vi "Connection.vi"(9 "전송":bool, 10 "데이터":string) -> ()   [LabVIEW 2020]
uses:
  <vilib>/Platform/TimedLoop/XDataNode/timing_clust.ctl
  <vilib>/Platform/TimedLoop/XDataNode/nitl_modes.ctl
  <vilib>/Platform/TimedLoop/XDataNode/wakeup.ctl
  WebSockets/WebSocket/WebSocket.lvclass/WebSocket.ctl
  WebSockets/WebSocket Server/WebSocket Server.lvclass/WebSocket Server.ctl
  WebSockets/WebSocket/Read Return Headers.vi
  WebSockets/WebSocket Server/Read Request URI.vi
  WebSockets/WebSocket Server/WebSocket Server.lvclass
  var.vi
  <vilib>/Platform/TimedLoop/XDataNode/XDataNode.xnode
  Sockets/VISA TCP Listener/VISA TCP Listener.lvclass
  <vilib>/Platform/TimedLoop/XDataNode/XDNodeRunTimeDep.lvlib
panel:
  out "데이터_자동":string
  in  "Stop":bool
  out "수신된 데이터":string
  out "HTTP Headers":variant
  out "Request URI":string
  # "소켓통신을 전담하는 subVI"
  # "2017243031 최주홍"
  # "수동으로 전송하는 용도"
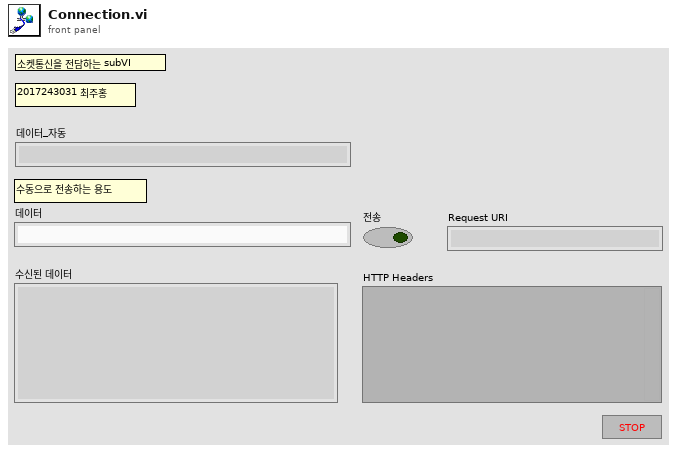
[diagram p1: front panel]
types:
  T1 = typedef "XDNodeRunTimeDep.lvlib/timing_clust.ctl" = cluster{"Expected End [f-1]":u64, "Actual End [f-1]":u64, "Finished Late? [f-1]":bool, "Expected End [i-1]":u64, "Actual End [i-1]":u64, "Finished Late? [i-1]":bool, "Expected Start [i]":u64, "Actual Start [i]":u64, "Expected Start [f]":u64, "Actual Start [f]":u64, "Source Name":string, "Structure Name":string, "Period":i64, "Deadline":i64, "Offset":i64, "Start":i64, "Priority":i32, "Timeout":i32, "Mode":T2, "Wakeup Reason":T3, "Error":errorcluster, "Source Type":string, "Secondary Source Type":string, "Global End Time":u64, "Global Start Time":u64, "Frame Duration":u64, "Iteration Duration":u64, "Assigned CPU":i32, "I/O Scan Engine Mode":u32}
  T2 = typedef "XDNodeRunTimeDep.lvlib/nitl_modes.ctl" = enum32{"No Change", "Process missed periods, maintain original phase", "Discard missed periods, maintain original phase", "Process missed periods, ignore original phase", "Discard missed periods, ignore original phase"}
  T3 = typedef "XDNodeRunTimeDep.lvlib/wakeup.ctl" = enum32{"Normal", "Aborted", "Asynchronous wakeup", "Timing source error", "Timed loop error", "Timeout"}
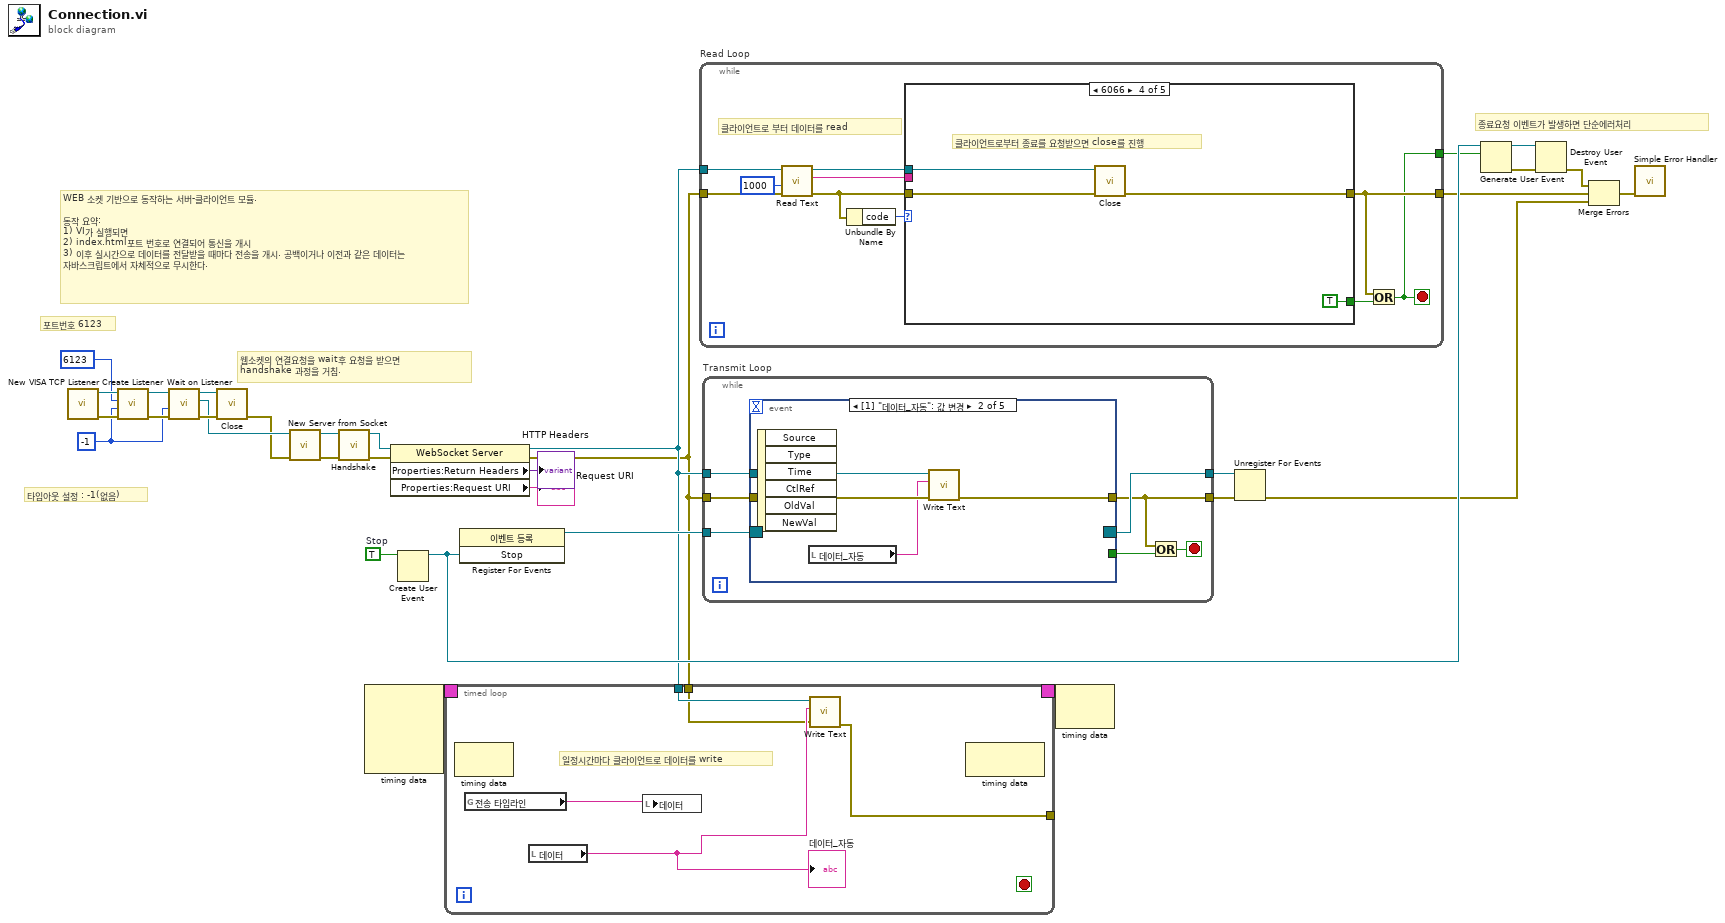
[diagram p0: block diagram]
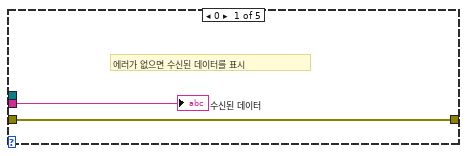
[diagram p2: hidden frame]
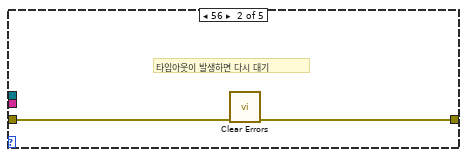
[diagram p3: hidden frame]
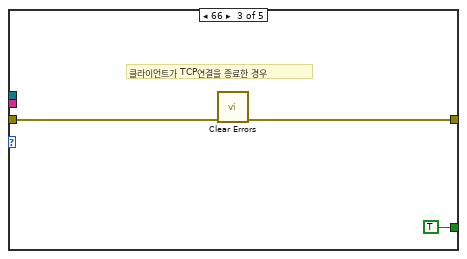
[diagram p4: hidden frame]
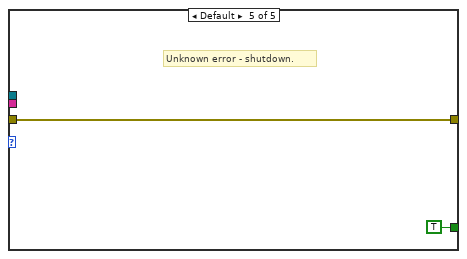
[diagram p5: hidden frame]
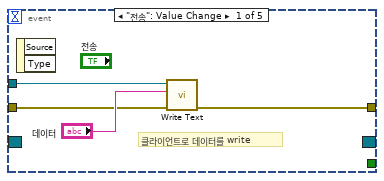
[diagram p6: hidden frame]
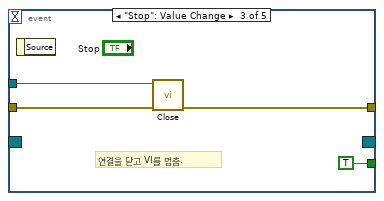
[diagram p7: hidden frame]
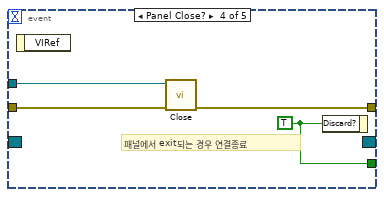
[diagram p8: hidden frame]
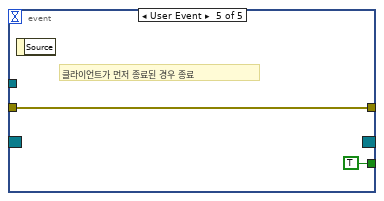
[diagram p9: hidden frame]
diagram:
  w31 = TRUE  # Stop
  w7 = -1 ("timeout ms (25000)")
  # "타임아웃 설정 : -1(없음)"
  # "종료요청 이벤트가 발생하면 단순에러처리"
  # "WEB 소켓 기반으로 동작하는 서버-클라이언트 모듈.\n\n동작 요약:\n1) VI가 실행되면\n2) index.html포트 번호로 연결되어 통신을 개시\n3) 이후 실시간으로 데이터를 전달받을 때마다 전송을 개시. 공백이거나 이전과 같은 데이터는 자바스크립트에서 자체적으로 무시한다."
  # "웹소켓의 연결요청을 wait후 요청을 받으면\nhandshake 과정을 거침."
  # "포트번호 6123"
  n1 = call "New VISA TCP Listener.vi"() -> ("error out"=w13:errorcluster, "VISA TCP Listener out"=w14:refnum<class "VISA TCP Listener.lvclass">)  [unwired: 10 in]
  n2 = call-dynamic "Create Listener.vi"("error in (no error)"=w13, "timeout ms (5000)"=w7, "Port"=u16 6123 ("port"), "VISA TCP Listener in"=w14) -> ("error out"=w11:errorcluster, "VISA TCP Listener out"=w9:refnum<class "VISA TCP Listener.lvclass">)  [unwired: 6 in]
  n3 = call-dynamic "Wait on Listener.vi"("error in (no error)"=w11, "timeout ms (5000)"=w7, "VISA TCP Listener in"=w9) -> ("error out"=w12:errorcluster, "Socket out"=w6:refnum<class "Socket.lvclass">, "VISA TCP Listener out"=w10:refnum<class "VISA TCP Listener.lvclass">)  [unwired: 6 in]
  n4 = call-dynamic "Close.vi"("error in (no error)"=w12, "VISA TCP Listener in"=w10) -> ("error out"=w5:errorcluster)  [unwired: 9 in]
  n5 = call "New Server from Socket.vi"("error in (no error)"=w5, "Socket"=w6) -> ("error out"=w18:errorcluster, "WebSocket Server out"=w19:refnum<class "WebSocket Server.lvclass">)  [unwired: 8 in]
  n6 = call-dynamic "Handshake.vi"("error in (no error)"=w18, "WebSocket Connection in"=w19) -> ("error out"=w20:errorcluster, "WebSocket Connection out"=w17:refnum<class "WebSocket Server.lvclass">)  [unwired: 8 in]
  n7 = node-c288() -> (w4:T1)  [unwired: 4 in]
  n8 = property class="WebSocket Server"(reference=w17, error in=w20) -> (reference out=w2:refnum<class "WebSocket Server.lvclass">, error out=w1:errorcluster, "Properties:Return Headers"=→"HTTP Headers":variant, "Properties:Request URI"=→"Request URI":string)
  n9 = Create User Event(user event datatype=w31) -> (user event=w29:refnum<user-event>)  [unwired: 1 in, 1 out]
  n10 = timed-loop {
    timing: w4 -> [_]
    timing-out: [_] -> w3
    tunnel: w2 -> [w35]
    tunnel: w1 -> [w34]
    tunnel: [w33] -> _
    stop <- _ stop-if-true
    # "일정시간마다 클라이언트로 데이터를 write"
    n11 = node-c288() -> ()  [unwired: 1 in, 1 out]
    n12 = global read "var.vi" "전송 타임라인"() -> (w37:string)
    n13 = local read "데이터"() -> (w36:string)
    "데이터_자동" <- w36
    n14 = local write "데이터"(w37) -> ()
    n15 = call-dynamic "Write Text.vi"("error in (no error)"=w34, "String Data"=w36, "WebSocket in"=w35) -> ("error out"=w33:errorcluster)  [unwired: 7 in, 1 out]
    n16 = node-c288() -> ()  [unwired: 1 in, 1 out]
  }
  n17 = register-events(w29) -> (reference out=w32:refnum<event-registration>)  [unwired: 2 in, 1 out]
  n18 = while "Read Loop" {
    tunnel: w2 -> [w49]
    tunnel: [w40] -> w28
    tunnel: [w42] -> w22
    tunnel: w1 -> [w43]
    stop <- w40 stop-if-true
    # "클라이언트로 부터 데이터를 read"
    n19 = call-dynamic "Read Text.vi"("error in (no error)"=w43, "timeout ms (5000)"=1000 ("timeout ms (25000)"), "WebSocket in"=w49) -> ("error out"=w44:errorcluster, "Data"=w46:string, "WebSocket out"=w45:refnum<class "WebSocket Server.lvclass">)  [unwired: 6 in]
    n20 = Unbundle By Name(w44) -> ("code"=w47:i32)
    n21 = case shown="6066" w47 {
      tunnel: w46 -> [w51 _ _ _ _]
      tunnel: [_ _ TRUE TRUE TRUE] -> w41
      tunnel: w45 -> [_ _ _ w60 _]
      tunnel: w44 -> [w50 w53 w55 w58 w61]
      tunnel: [w50 w52 w54 w57 w61] -> w42
      frame 0 {
        # "에러가 없으면 수신된 데이터를 표시"
        "수신된 데이터" <- w51
      }
      frame 56 {
        # "타임아웃이 발생하면 다시 대기"
        n22 = call <vilib>:"Clear Errors.vi"("error in (no error)"=w53) -> ("error out"=w52:errorcluster)  [unwired: 5 in, 1 out]
      }
      frame 66 {
        # "클라이언트가 TCP연결을 종료한 경우"
        n23 = call <vilib>:"Clear Errors.vi"("error in (no error)"=w55) -> ("error out"=w54:errorcluster)  [unwired: 5 in, 1 out]
      }
      frame 6066 {
        # "클라이언트로부터 종료를 요청받으면 close를 진행"
        n24 = call-dynamic "Close.vi"("error in (no error)"=w58, "WebSocket in"=w60) -> ("error out"=w57:errorcluster)  [unwired: 9 in]
      }
      frame Default {
        # "Unknown error - shutdown."
      }
    }
    n25 = Or(x=w42, y=w41) -> (x .or. y?=w40:bool)
  }
  n26 = while "Transmit Loop" {
    tunnel: w2 -> [w69]
    tunnel: w32 -> [w68]
    tunnel: [w67] -> w30
    tunnel: [w63] -> w23
    tunnel: w1 -> [w66]
    stop <- w64 stop-if-true
    n27 = event shown="[1] \"데이터_자동\": 값 변경" {
      selector: w68 -> [_ _ _ _ _]
      dyn-events: [_ _ _ _ _] -> w67
      timeout: _ -> [_ _ _ _ _]
      tunnel: w69 -> [w73 w77 w80 w85 _]
      tunnel: [_ _ TRUE w84 TRUE] -> w65
      tunnel: [w70 w75 w79 w83 w86] -> w63
      tunnel: w66 -> [w71 w76 w78 w82 w86]
      event "전송": Value Change {
        # "클라이언트로 데이터를 write"
        n28 = event-data() -> ()  [unwired: 1 in, 2 out]
        n29 = call-dynamic "Write Text.vi"("error in (no error)"=w71, "String Data"="데이터", "WebSocket in"=w73) -> ("error out"=w70:errorcluster)  [unwired: 7 in, 1 out]
      }
      event "데이터_자동": Value Change {
        n30 = event-data() -> ()  [unwired: 1 in, 6 out]
        n31 = local read "데이터_자동"() -> (w74:string)
        n32 = call-dynamic "Write Text.vi"("error in (no error)"=w76, "String Data"=w74, "WebSocket in"=w77) -> ("error out"=w75:errorcluster)  [unwired: 7 in, 1 out]
      }
      event "Stop": Value Change {
        # "연결을 닫고 VI를 멈춤."
        n33 = event-data() -> ()  [unwired: 1 in, 1 out]
        n34 = call-dynamic "Close.vi"("error in (no error)"=w78, "WebSocket in"=w80) -> ("error out"=w79:errorcluster)  [unwired: 9 in]
      }
      event Panel Close? {
        w84 = TRUE ("Discard?")
        # "패널에서 exit되는 경우 연결종료"
        n35 = event-data() -> ()  [unwired: 1 in, 1 out]
        n36 = call-dynamic "Close.vi"("error in (no error)"=w82, "WebSocket in"=w85) -> ("error out"=w83:errorcluster)  [unwired: 9 in]
        n37 = event-data("Discard?"=w84) -> ()  [unwired: 1 in, 1 out]
      }
      event User Event {
        # "클라이언트가 먼저 종료된 경우 종료"
        n38 = event-data() -> ()  [unwired: 1 in, 1 out]
      }
    }
    n39 = Or(x=w63, y=w65) -> (x .or. y?=w64:bool)
  }
  n40 = node-c288(w3) -> ()  [unwired: 1 out]
  n41 = Unregister For Events(event registration refnum=w30, error in=w23) -> (error out=w21:errorcluster)
  n42 = Generate User Event(user event=w29, event data cluster=w28) -> (user event out=w27:refnum<user-event>, error out=w26:errorcluster)  [unwired: 2 in]
  n43 = Destroy User Event(user event=w27, error in=w26) -> (error out=w25:errorcluster)
  n44 = Merge Errors(w25, w22, w21) -> (w24:errorcluster)
  n45 = call <vilib>:"Simple Error Handler.vi"("error in (no error)"=w24) -> ()  [unwired: 4 in, 5 out]
